vi "BRig_FPGA_triggerSolenoid.vi"(5 "input_Solenoid_MTrig":bool, 7 "input_Solenoid_trig":bool, 8 "input_threshold":u32, 10 "input_counter":u32, 11 "input_trig":bool) -> (0 "output_Solenoid_OnOff":bool, 2 "output_counter":u32, 3 "output_trig":bool)   [LabVIEW 2014]
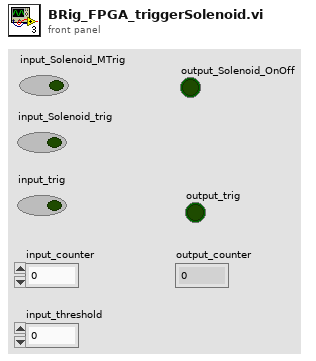
[diagram p1: front panel]
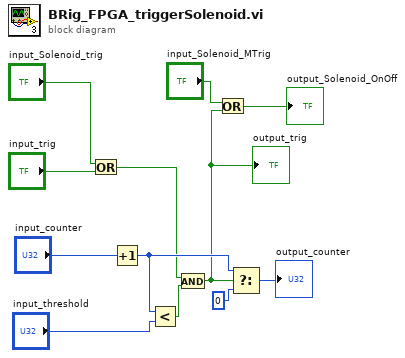
[diagram p0: block diagram]
diagram:
  n1 = Or(x="input_Solenoid_trig", y="input_trig") -> (x .or. y?=w5:bool)
  n2 = Increment(x="input_counter") -> (x+1=w7:u32)
  n3 = Less?(x=w7, y="input_threshold") -> (x < y?=w6:bool)
  n4 = And(x=w5, y=w6) -> (x .and. y?=w2:bool)
  "output_trig" <- w2
  n5 = Or(x="input_Solenoid_MTrig", y=w2) -> (x .or. y?=→"output_Solenoid_OnOff":bool)
  n6 = Select(t=w7, s=w2, f=u32 0) -> (s? t:f=→"output_counter":u32)
